vi "Read Sound ConfigurationI.vi"(8 "error constant":errorcluster, 11 "data value reference":refnum<data-value>) -> (0 "error out":errorcluster, 3 "Sound Manager Config":T1)   [LabVIEW 2021]
doc: "This method extracts is a Poliphormic method used to read each module configuration."
uses:
  Application/App Configuration.ctl
  Typedefs/Config.ctl
  Application/Application.lvclass
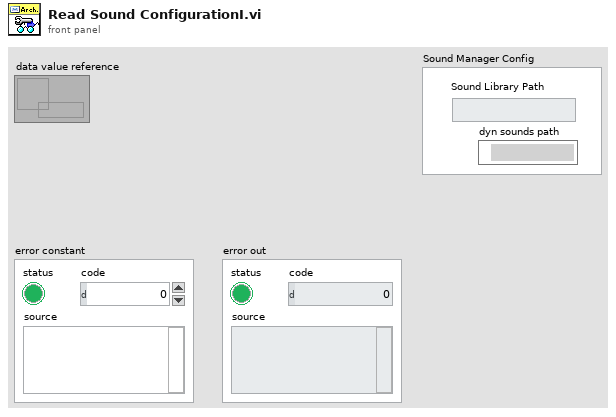
[diagram p1: front panel]
types:
  T1 = typedef "Config.ctl" = cluster{"Sound Library Path":path, "dyn sounds path":path}
  T2 = typedef "Application.lvclass/App Configuration.ctl" = cluster{"Sound Manager Config":T1}
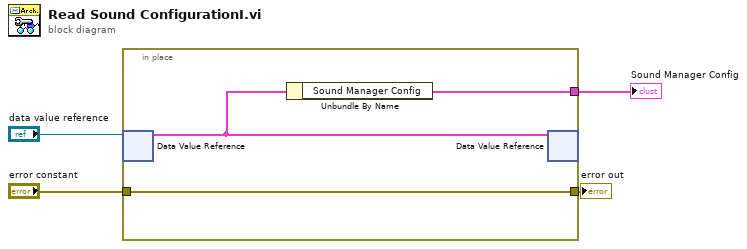
[diagram p0: block diagram]
diagram:
  n1 = in-place {
    in-place-border: [w5] -> w1
    in-place-border: "error constant" -> [w6]
    in-place-border: [w6] -> w2
    n2 = in-place-dvr #1("data value reference") -> (w7:T2)  [unwired: 1 out]
    n3 = Unbundle By Name(w7) -> ("Sound Manager Config"=w5:T1)
    n4 = in-place-dvr #1(w7) -> ()  [unwired: 2 out]
  }
  "error out" <- w2
  "Sound Manager Config" <- w1
